vi "Servos.vi"(8 "Error In":errorcluster, 9 "Pulse Widths (uS)":u16[](array[numeric]), 10 "Servo Channels 2":u8[](array[numeric]), 11 "LINX Resource":T1) -> (0 "Error Out":errorcluster, 3 "LINX Resource":T1)   [LabVIEW 2018]
uses:
  <vilib>/MakerHub/LINX/Public/Sensors/Motion/Servo/Servo.lvlib
  <vilib>/MakerHub/LINX/Public/Sensors/Motion/Servo/Servo Set Pulse Width N Channels.vi
  <vilib>/MakerHub/LINX/Private/Type Defs/Platform.ctl
  <vilib>/MakerHub/LINX/LMH-LINX.lvlib
  <vilib>/MakerHub/LINX/Private/Type Defs/Interface.ctl
  <vilib>/MakerHub/LINX/Private/Device/Type Defs/TCP Config.ctl
  <vilib>/MakerHub/LINX/Private/Device/Device.lvlib
  <vilib>/MakerHub/LINX/Private/Device/Type Defs/Channels.ctl
  <vilib>/MakerHub/LINX/Private/Device/Type Defs/LINX Device Config.ctl
  <vilib>/MakerHub/LINX/Private/Type Defs/LINX Ref.ctl
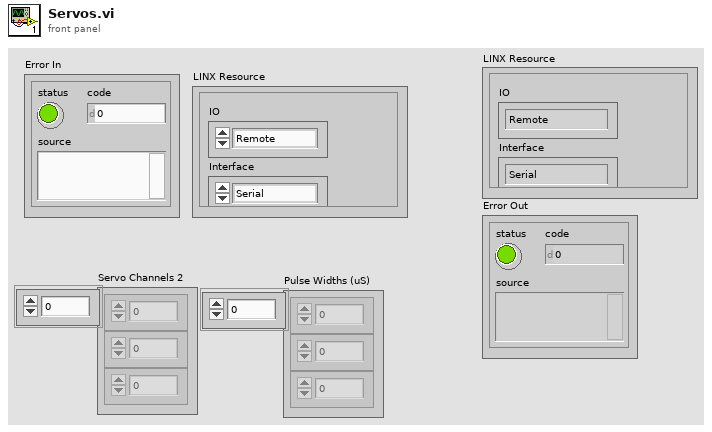
[diagram p1: front panel]
types:
  T1 = typedef "LMH-LINX.lvlib/LINX Ref.ctl" = cluster{"IO":T2, "Interface":T3, "LINX Device Config":T4}
  T2 = typedef "LMH-LINX.lvlib/Platform.ctl" = enum16{"Remote", "Local"}
  T3 = typedef "LMH-LINX.lvlib/Interface.ctl" = enum16{"Serial", "TCP"}
  T4 = typedef "LMH-LINX.lvlib/Device.lvlib/LINX Device Config.ctl" = cluster{"Interface":T3, "COM Port":refnum<visa-resource-name>, "TCP Configuration":T5, "Device Family":u8, "Device ID":u8, "Device Name":string, "TCP Ref":refnum<k5>, "Channels":T6}
  T5 = typedef "LMH-LINX.lvlib/Device.lvlib/TCP Config.ctl" = cluster{"IP Address":string, "Port":u16}
  T6 = typedef "LMH-LINX.lvlib/Channels.ctl" = cluster{"DI":u8[], "DO":u8[], "AI":u8[], "AO":u8[], "PWM":u8[], "QE":u8[], "UART":u8[], "I2C 2":u8[], "SPI":u8[], "CAN":u8[], "Servo":u8[], "AI Ref (V)":dbl, "AI Resolution (Bits)":u8, "AO Ref (V)":dbl, "AO Resolution (Bits)":u8}
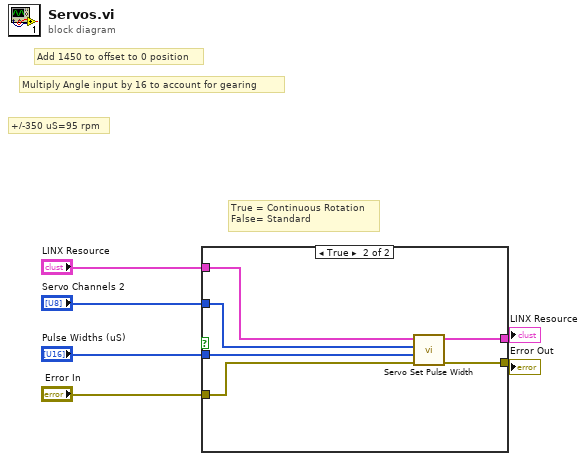
[diagram p0: block diagram]
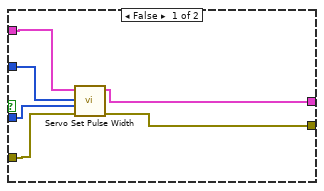
[diagram p2: hidden frame]
diagram:
  # "True = Continuous Rotation\nFalse= Standard"
  # "Add 1450 to offset to 0 position"
  # "Multiply Angle input by 16 to account for gearing"
  # "+/-350 uS=95 rpm"
  n1 = case shown="True" {
    selector: _ -> [_ _]
    tunnel: "Servo Channels 2" -> [w11 w18]
    tunnel: "LINX Resource" -> [w12 w17]
    tunnel: "Pulse Widths (uS)" -> [w10 w16]
    tunnel: "Error In" -> [w9 w15]
    tunnel: [w7 w14] -> w2
    tunnel: [w8 w13] -> w1
    frame False {
      n2 = call-poly <vilib>:"Servo Set Pulse Width.vi"("Error In"=w9, "Pulse Widths (uS)"=w10, "Servo Channels"=w11, "LINX Resource"=w12) -> ("Error Out"=w8:errorcluster, "LINX Resource"=w7:T1)  [unwired: 6 in]
    }
    frame True {
      n3 = call-poly <vilib>:"Servo Set Pulse Width.vi"("Error In"=w15, "Pulse Widths (uS)"=w16, "Servo Channels"=w18, "LINX Resource"=w17) -> ("Error Out"=w13:errorcluster, "LINX Resource"=w14:T1)  [unwired: 6 in]
    }
  }
  "LINX Resource" <- w2
  "Error Out" <- w1
